vi "MSEncoder Case-10-UpdRFChBias.vi"(8 "error in (no error)":errorcluster, 9 "ParamValIn":variant, 11 "MSEncoder in":refnum<class "MSEncoder.lvclass">) -> (0 "error out":errorcluster, 3 "MSEncoder out":refnum<class "MSEncoder.lvclass">)   [LabVIEW 2018, in "MSEncoder.lvclass"]
uses:
  MSEncoder.lvclass
  Ctl/MSEditorParam updRFBias.ctl
  MSEncoder.lvclass/MSEncoder.ctl
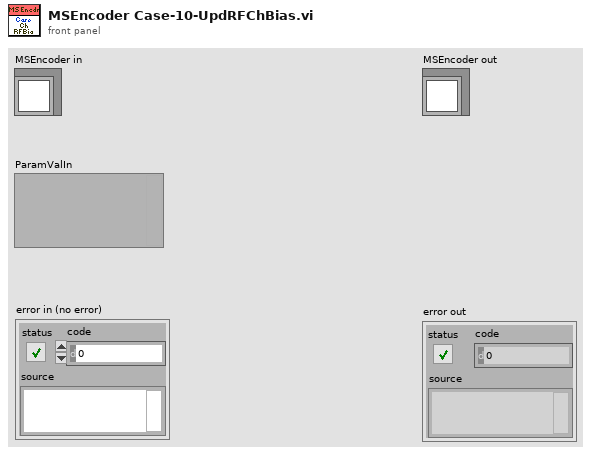
[diagram p1: front panel]
types:
  T1 = typedef "MSEditorParam updRFBias.ctl" = cluster{"ch1":dbl, "ch2":dbl, "ch3":dbl}
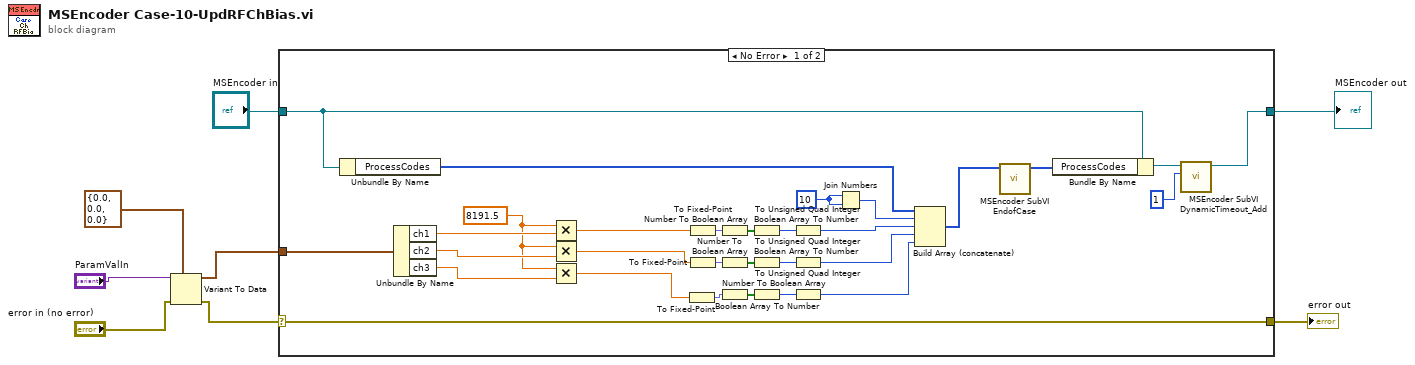
[diagram p0: block diagram]
diagram:
  n1 = Variant To Data(error in="error in (no error)", type=T1 {"ch1"=0.0, "ch2"=0.0, "ch3"=0.0} ("ParamValueType"), Variant="ParamValIn") -> (data=w3:T1, error out=w2:errorcluster)
  n2 = case shown="No Error" w2 {
    selector: w2 -> [w32 w40]
    tunnel: "MSEncoder in" -> [w37 w39]
    tunnel: [w32 w40] -> w8
    tunnel: [w25 w39] -> w7
    tunnel: w3 -> [w31 _]
    frame No Error {
      w20 = 8191.5 ("y")
      w35 = u32 10
      n3 = Unbundle By Name(w37) -> ("ProcessCodes"=w38:u64[])
      n4 = Unbundle By Name(w31) -> ("ch1"=w30:dbl, "ch2"=w22:dbl, "ch3"=w21:dbl)
      n5 = Multiply(x=w20, y=w30) -> (x*y=w29:dbl)
      n6 = Multiply(x=w20, y=w22) -> (x*y=w12:dbl)
      n7 = Multiply(x=w20, y=w21) -> (x*y=w11:dbl)
      n8 = To Fixed-Point(number=w11) -> (fixed-point=w15:fxp<+/-,16,14>)  [unwired: 1 in]
      n9 = To Fixed-Point(number=w29) -> (fixed-point=w16:fxp<+/-,16,14>)  [unwired: 1 in]
      n10 = To Fixed-Point(number=w12) -> (fixed-point=w17:fxp<+/-,16,14>)  [unwired: 1 in]
      n11 = Number To Boolean Array(number=w16) -> (Boolean array=w23:bool[])
      n12 = Number To Boolean Array(number=w17) -> (Boolean array=w19:bool[])
      n13 = Number To Boolean Array(number=w15) -> (Boolean array=w13:bool[])
      n14 = Boolean Array To Number(Boolean array=w23) -> (number=w28:u16)
      n15 = Boolean Array To Number(Boolean array=w19) -> (number=w18:u16)
      n16 = Boolean Array To Number(Boolean array=w13) -> (number=w14:u16)
      n17 = To Unsigned Quad Integer(1:w28) -> (0:w27:u64)
      n18 = To Unsigned Quad Integer(1:w18) -> (0:w10:u64)
      n19 = To Unsigned Quad Integer(1:w14) -> (0:w9:u64)
      n20 = Join Numbers(hi=w35, lo=w35) -> ((hi.lo)=w34:u64)
      n21 = Build Array (concatenate)(w38, w34, w27, w10, w9) -> (w33:u64[])
      n22 = call "MSEncoder SubVI EndofCase.vi"("Case codes"=w33) -> ("Case codes with end"=w36:u64[])  [unwired: 9 in, 1 out]
      n23 = Bundle By Name(cluster=w37, "ProcessCodes"=w36) -> (w26:refnum<class "MSEncoder.lvclass">)
      n24 = call "MSEncoder SubVI DynamicTimeout_Add.vi"("Timeout_ms"=1, "MSEncoder"=w26) -> ("MSEncoder"=w25:refnum<class "MSEncoder.lvclass">)  [unwired: 8 in, 1 out]
    }
    frame Error {
    }
  }
  "error out" <- w8
  "MSEncoder out" <- w7
